vi "UTF8 String to JSON.vi"(9 "error in (no error)":errorcluster, 11 "UTF8 String":string) -> (1 "error out":errorcluster, 3 "<JSON>":string)   [LabVIEW 2021, in "json.facade.lvlib"]
doc: "Converts a UTF-8 encoded string into a JSON String value. \n\nNote that the regular \"To JSON\" function assumes strings are in System encoding. This function is to allow working with UTF-8 encoded text in LabVIEW."
uses:
  json.facade.lvlib
  jsontext/JSONtext.lvlib
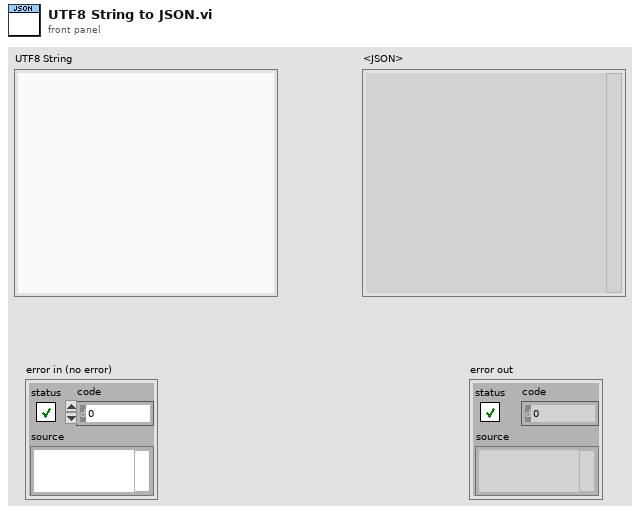
[diagram p1: front panel]
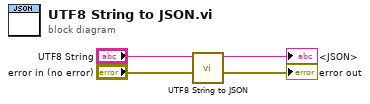
[diagram p0: block diagram]
diagram:
  n1 = call "UTF8 String to JSON.vi"("error in (no error)"="error in (no error)", "UTF8 String"="UTF8 String") -> ("error out"=→"error out":errorcluster, "<JSON>"=→"<JSON>":string)  [unwired: 8 in]
